vi "Main.vi"() -> ()   [LabVIEW 2021]
uses:
  <vilib>/DAQmx/write.llb/DAQmx Write (Digital Bool 1Line 1Point).vi
  <vilib>/Utility/file.llb/Write Delimited Spreadsheet (DBL).vi
  <vilib>/DAQmx/miscellaneous.llb/DAQmx Fill In Error Info.vi
panel:
  in  "T-Minus Control":dbl=2.0
  out "Ignition":bool
  out "T-Minus 10":dbl(slide) scale=0.0..30.0
  out "Run Time":dbl=5.0 caption="Time Target (s)"
  out "Recording":bool
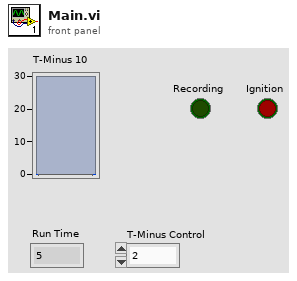
[diagram p1: front panel]
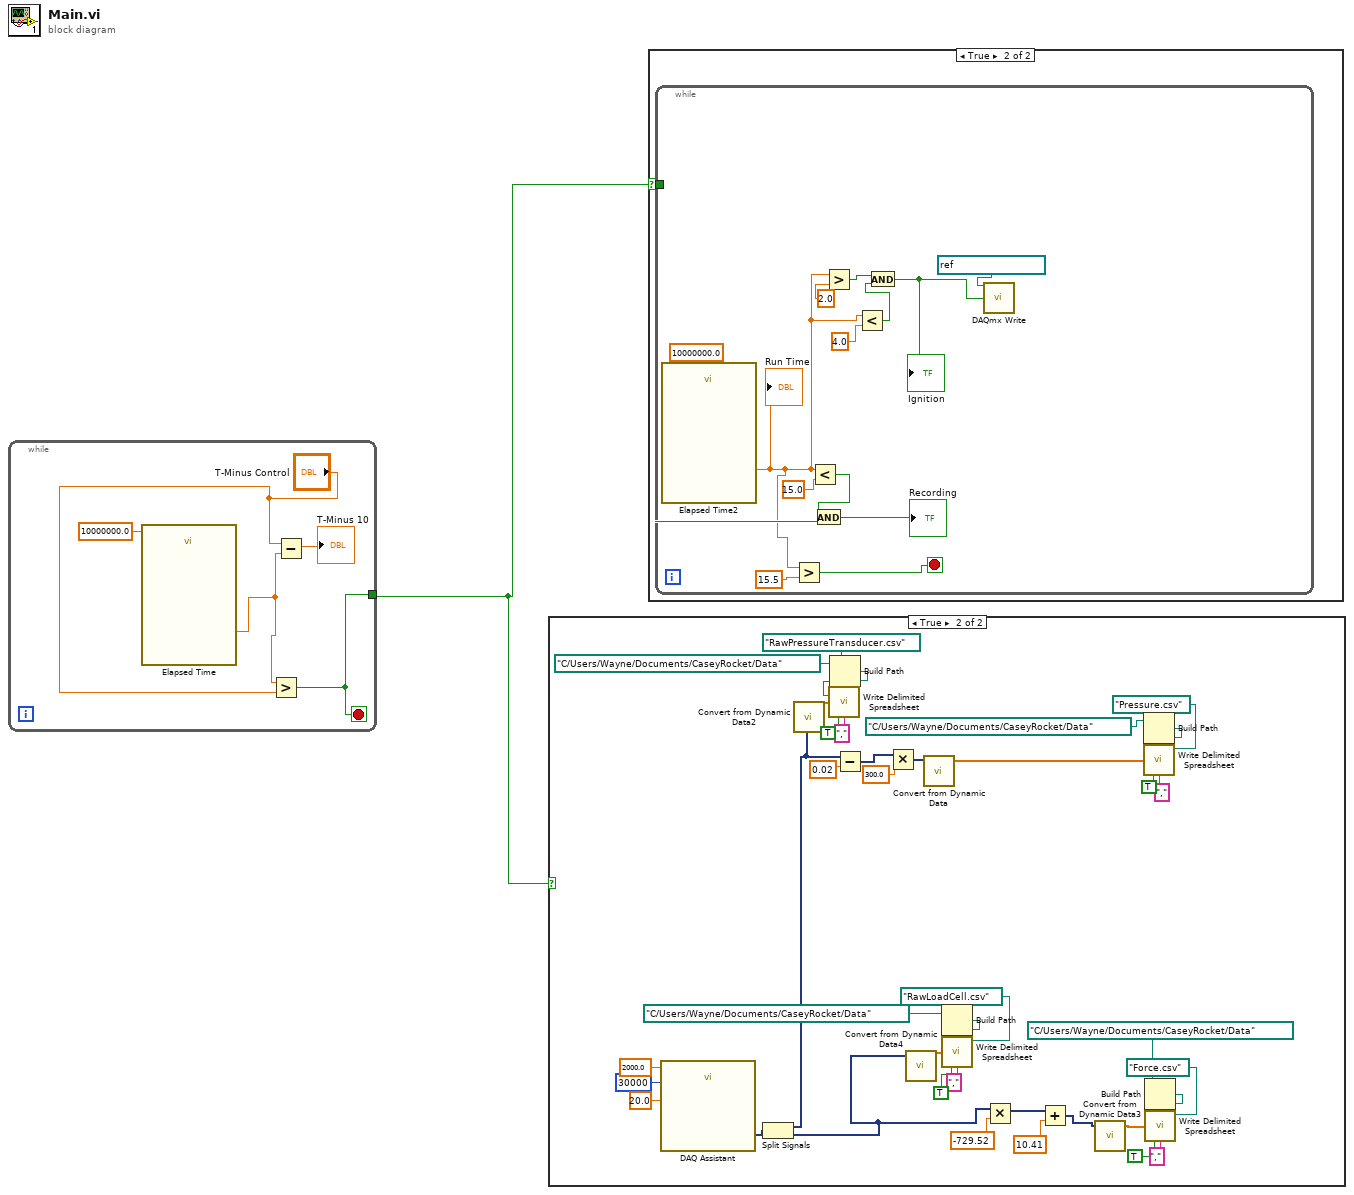
[diagram p0: block diagram]
diagram:
  n1 = while {
    tunnel: [w5] -> w1
    stop <- w5 stop-if-true
    n2 = call "Elapsed Time"("Time Target (s)"=10000000.0) -> ("Elapsed Time (s)"=w4:dbl)  [unwired: 11 in, 7 out]
    n3 = Greater?(x=w4, y="T-Minus Control") -> (0:w5:bool)
    n4 = Subtract(x="T-Minus Control", y=w4) -> (x-y=→"T-Minus 10":dbl)
  }
  n5 = case shown="True" w1 {
    frame False {
    }
    frame True {
      n6 = call "DAQ Assistant"("rate"=2000.0, "number of samples"=30000, "timeout (s)"=20.0) -> ("data"=w34:dynamicdata)  [unwired: 14 in, 2 out]
      n7 = Split Signals(w34) -> (w33:dynamicdata, w22:dynamicdata)  [unwired: 2 in]
      n8 = call "Convert from Dynamic Data2"("Dynamic Data Type"=w33) -> ("Array"=w38:dbl[])  [unwired: 3 in]
      n9 = Build Path(base path=path "C:/Users/Wayne/Documents/CaseyRocket/Data", name or relative path=path "RawPressureTransducer.csv") -> (appended path=w39:path)
      n10 = call-poly <vilib>:"Write Delimited Spreadsheet.vi"("file path (dialog if empty)"=w39, "1D data"=w38, "transpose? (no:F)"=TRUE, "delimiter (\\t)"="," ("delimiter (\\t)")) -> ()  [unwired: 10 in, 2 out]
      n11 = Subtract(x=w33, y=0.02) -> (x-y=w35:dynamicdata)
      n12 = Multiply(x=w35, y=300.0) -> (x*y=w21:dynamicdata)
      n13 = call "Convert from Dynamic Data4"("Dynamic Data Type"=w22) -> ("Array"=w27:dbl[])  [unwired: 3 in]
      n14 = call "Convert from Dynamic Data"("Dynamic Data Type"=w21) -> ("Array"=w20:dbl[])  [unwired: 3 in]
      n15 = Build Path(base path=path "C:/Users/Wayne/Documents/CaseyRocket/Data", name or relative path=path "RawLoadCell.csv") -> (appended path=w28:path)
      n16 = call-poly <vilib>:"Write Delimited Spreadsheet.vi"("file path (dialog if empty)"=w28, "1D data"=w27, "transpose? (no:F)"=TRUE, "delimiter (\\t)"="," ("delimiter (\\t)")) -> ()  [unwired: 10 in, 2 out]
      n17 = Multiply(x=w22, y=-729.52) -> (x*y=w24:dynamicdata)
      n18 = Add(x=w24, y=10.41) -> (x+y=w23:dynamicdata)
      n19 = call "Convert from Dynamic Data3"("Dynamic Data Type"=w23) -> ("Array"=w18:dbl[])  [unwired: 3 in]
      n20 = Build Path(base path=path "C:/Users/Wayne/Documents/CaseyRocket/Data", name or relative path=path "Pressure.csv") -> (appended path=w42:path)
      n21 = call-poly <vilib>:"Write Delimited Spreadsheet.vi"("file path (dialog if empty)"=w42, "1D data"=w20, "transpose? (no:F)"=TRUE, "delimiter (\\t)"="," ("delimiter (\\t)")) -> ()  [unwired: 10 in, 2 out]
      n22 = Build Path(base path=path "C:/Users/Wayne/Documents/CaseyRocket/Data", name or relative path=path "Force.csv") -> (appended path=w30:path)
      n23 = call-poly <vilib>:"Write Delimited Spreadsheet.vi"("file path (dialog if empty)"=w30, "1D data"=w18, "transpose? (no:F)"=TRUE, "delimiter (\\t)"="," ("delimiter (\\t)")) -> ()  [unwired: 10 in, 2 out]
    }
  }
  n24 = case shown="True" w1 {
    selector: w1 -> [_ w45]
    frame False {
    }
    frame True {
      n25 = while {
        tunnel: w45 -> [w58]
        stop <- w53 stop-if-true
        n26 = call "Elapsed Time2"("Time Target (s)"=10000000.0) -> ("Elapsed Time (s)"=w48:dbl)  [unwired: 11 in, 7 out]
        "Run Time" <- w48
        n27 = Greater?(x=w48, y=15.5) -> (0:w53:bool)
        n28 = Less?(x=w48, y=15.0) -> (x < y?=w57:bool)
        n29 = And(x=w57, y=w58) -> (x .and. y?=→"Recording":bool)
        n30 = Greater?(x=w48, y=2.0) -> (0:w50:bool)
        n31 = Less?(x=w48, y=4.0) -> (x < y?=w49:bool)
        n32 = And(x=w50, y=w49) -> (x .and. y?=w46:bool)
        "Ignition" <- w46
        n33 = call-poly <vilib>:"DAQmx Write.vi"("task/channels in"=refnum<k21> "Rocket Ignition", "data"=w46) -> ()  [unwired: 11 in, 3 out]
      }
    }
  }
